vi "Constants.vi"() -> ()   [LabVIEW 2018, in "Displacement Measurement CD Shared.lvlib"]
doc: "Use this Global VI to access the GUIDs assigned to the page resources of the Custom Device."
uses:
  Displacement Measurement CD Shared.lvlib
panel:
  in  "Tab Control":enum32{"GUIDS", "Constants", "Properties"}(tab)
  in  "Displacement Measurement CD":string="8ca23031-31bf-47ef-8851-ce8a975a3958"
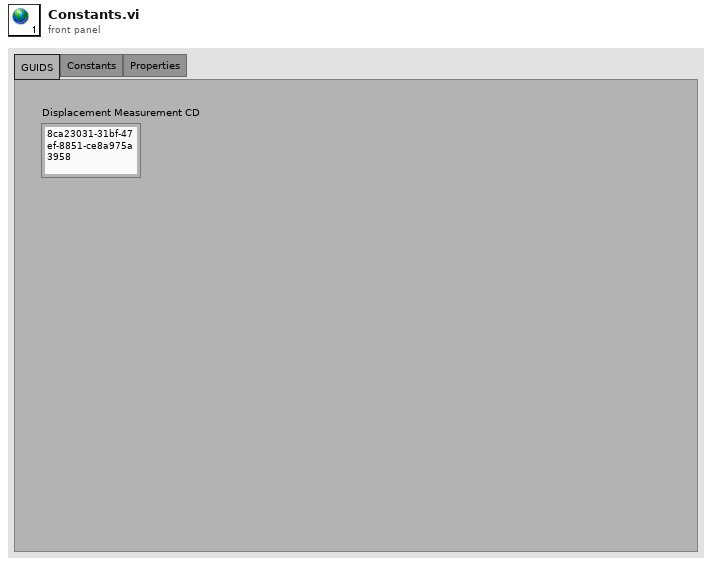
[diagram p1: front panel]
diagram:
